vi "Write Named Numeric Size Width.vi"(8 "error in (no error)":errorcluster, 10 "Width":u32, 11 "NamedNumeric.lvclass in":refnum<class "NamedNumeric.lvclass">) -> (0 "error out":errorcluster, 3 "NamedNumeric.lvclass out":refnum<class "NamedNumeric.lvclass">)   [LabVIEW 2015, in "NamedNumeric.lvclass"]
uses:
  NamedNumeric.lvclass
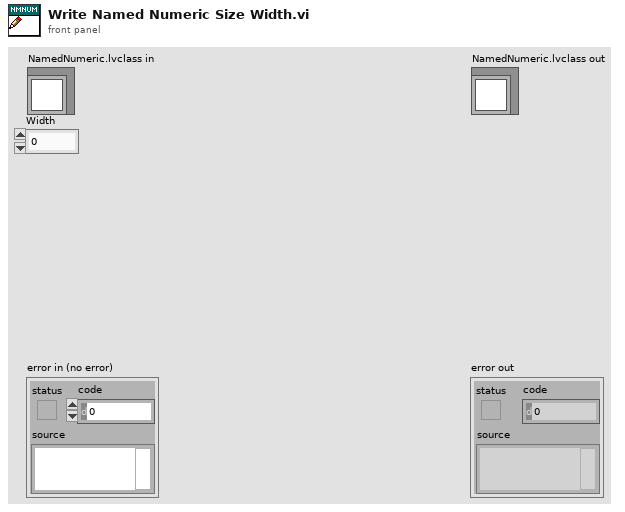
[diagram p1: front panel]
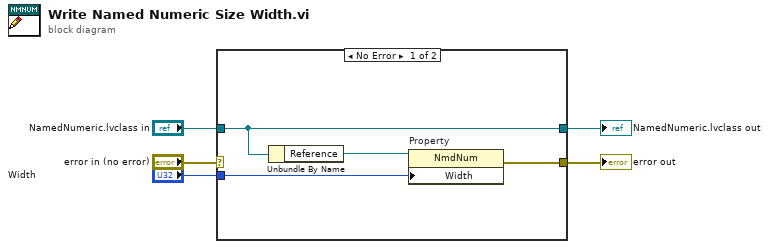
[diagram p0: block diagram]
diagram:
  n1 = case shown="No Error" "error in (no error)" {
    selector: "error in (no error)" -> [_ w11]
    tunnel: [w9 w11] -> w4
    tunnel: [w7 w10] -> w2
    tunnel: "NamedNumeric.lvclass in" -> [w7 w10]
    tunnel: "Width" -> [w8 _]
    frame No Error {
      n2 = Unbundle By Name(w7) -> ("Reference"=w6:refnum<vi>)
      n3 = property on="Property" class="NmdNum"(reference=w6, "Width"=w8) -> (error out=w9:errorcluster)  [unwired: 1 in, 1 out]
    }
    frame Error {
    }
  }
  "error out" <- w4
  "NamedNumeric.lvclass out" <- w2
